vi "stopDAQ.vi"(8 "error in (no error)":errorcluster, 11 "Instrument.Lockin in":refnum<class "Instrument.Lockin.lvclass">) -> (0 "error out":errorcluster, 3 "Instrument.Lockin out":refnum<class "Instrument.Lockin.lvclass">)   [LabVIEW 2019, in "Instrument.Lockin.lvlib" / "Instrument.Lockin.lvclass"]
doc: "Stop acquiring data..\n\nIf address=\"\", this API reads from localhost\nIf address is remote lockin, you need to add this computer to allowed whitelist on the lockin computer you are trying to access."
uses:
  Instrument.Lockin.lvclass
  <userlib>/LevyLab/Instrument Framework/Instrument Types/Lockin/Instrument.LockinAPI.lvclass
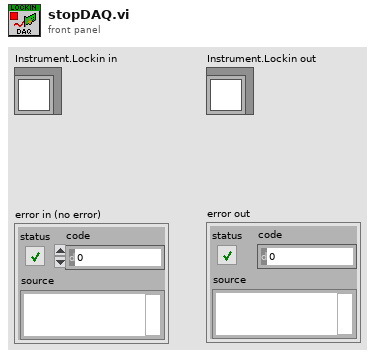
[diagram p1: front panel]
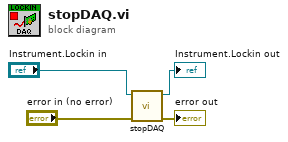
[diagram p0: block diagram]
diagram:
  n1 = call-parent "stopDAQ.vi"("error in (no error)"="error in (no error)", "Instrument.LockinAPI in"="Instrument.Lockin in") -> ("error out"=→"error out":errorcluster, "Instrument.LockinAPI out"=→"Instrument.Lockin out":refnum<class "Instrument.Lockin.lvclass">)  [unwired: 8 in]
